vi "createPath.vi"(8 "error in (no error)":errorcluster, 10 "filename":string, 11 "Settings in":refnum<class "Settings.lvclass">) -> (0 "error out":errorcluster, 2 "Path":path, 3 "Settings out":refnum<class "Settings.lvclass">)   [LabVIEW 2016, in "Settings.lvclass"]
uses:
  Settings.lvclass
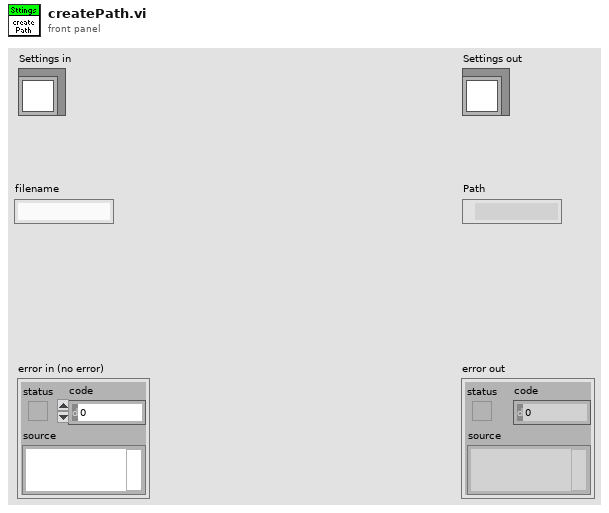
[diagram p1: front panel]
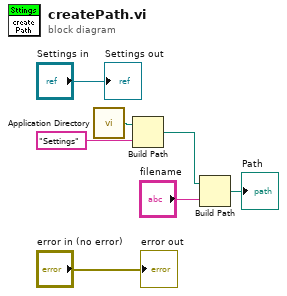
[diagram p0: block diagram]
diagram:
  n1 = call <vilib>:"Application Directory.vi"() -> ("Application Directory"=w5:path)
  n2 = Build Path(base path=w5, name or relative path="Settings") -> (appended path=w2:path)
  n3 = Build Path(base path=w2, name or relative path="filename") -> (appended path=→"Path":path)
  "error out" <- "error in (no error)"
  "Settings out" <- "Settings in"
